vi "Stop Core.vi"(10 "final error code":i32, 11 "Limites Contador in":refnum<class "Limites Contador.lvclass">) -> (3 "Limites Contador out":refnum<class "Limites Contador.lvclass">)   [LabVIEW 2020, in "Limites Contador.lvlib" / "Limites Contador.lvclass"]
doc: "(<B>Filename</B>: Actor Framework.lvlib:Actor.lvclass:Stop Core.vi)\n\nDefines what the actor does before it stops. Use the <B>final error code</B> input to determine whether the actor shut down in response to an error.\n\nBy default, this method passes the Stop message along to all auto-stop nested actors. A descendant class may override this method to define additional behavior, such as shutting down any processes the actor initiated in its override of the Actor Core method."
uses:
  Limites Contador.lvclass
  <vilib>/ActorFramework/Actor/Actor.lvclass
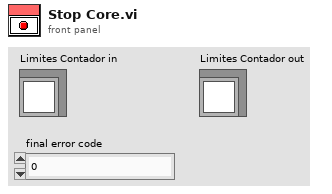
[diagram p1: front panel]
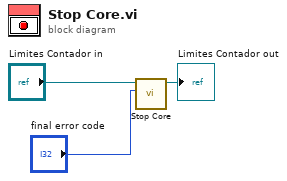
[diagram p0: block diagram]
diagram:
  n1 = call-parent "Stop Core.vi"("final error code"="final error code", "Actor in"="Limites Contador in") -> ("Actor out"=→"Limites Contador out":refnum<class "Limites Contador.lvclass">)  [unwired: 9 in]
